vi "ReadMsgs.vi"(0 "reference in":refnum<class "MessageInterface.lvclass">, 11 "error in (no error)":errorcluster) -> (4 "reference out":refnum<class "MessageInterface.lvclass">, 6 "msgs":T1[](array[typedef]), 15 "error out":errorcluster)   [LabVIEW 2019, in "MessageInterface.lvclass"]
uses:
  MessageInterface.lvclass
  Message.ctl
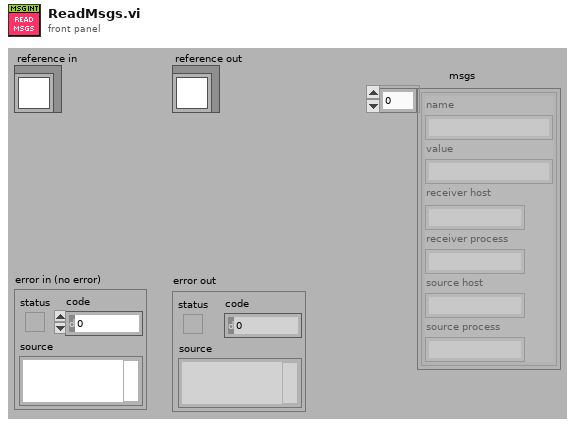
[diagram p1: front panel]
types:
  T1 = typedef "MessageInterface.lvclass/Message.ctl" = cluster{"name":string, "value":string, "receiver host":string, "receiver process":string, "source host":string, "source process":string}
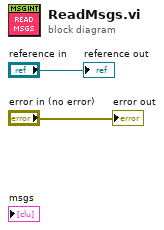
[diagram p0: block diagram]
diagram:
  "error out" <- "error in (no error)"
  "reference out" <- "reference in"
